vi "U3 PWM16.vi"(8 "error in":errorcluster, 9 "PWM Duty Cycle [%]":dbl=50.0 format="%.4f") -> (0 "error out":errorcluster)   [LabVIEW 2021]
panel:
  out "aTimerValues":u16[](array[numeric])
  in  "FirstFound":bool=TRUE
  in  "Address":string="1"
  out "Error Message":string
  # "Demonstrates 1 timer channel of 16-bit PWM output on FIO4 with a frequency of 40.7 Hz."
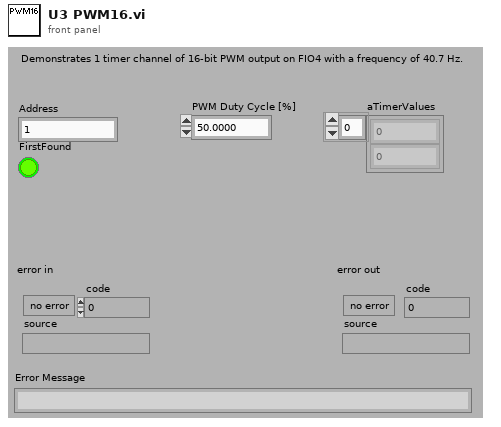
[diagram p1: front panel]
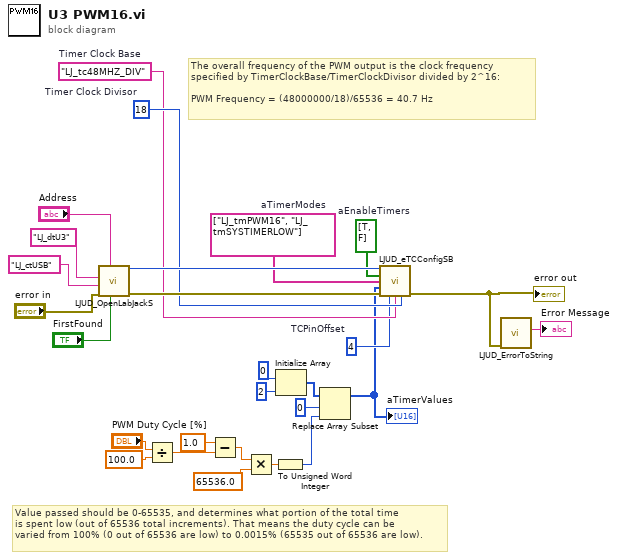
[diagram p0: block diagram]
diagram:
  w4 = 4  # TCPinOffset
  w3 = bool[] [TRUE, FALSE]  # aEnableTimers
  w6 = 18  # Timer Clock Divisor
  w5 = "LJ_tc48MHZ_DIV"  # Timer Clock Base
  w7 = string[] ["LJ_tmPWM16", "LJ_tmSYSTIMERLOW"]  # aTimerModes
  # "The overall frequency of the PWM output is the clock frequency\nspecified by TimerClockBase/TimerClockDivisor divided by 2^16:\n\nPWM Frequency = (48000000/18)/65536 = 40.7 Hz"
  # "Value passed should be 0-65535, and determines what portion of the total time\nis spent low (out of 65536 total increments). That means the duty cycle can be\nvaried from 100% (0 out of 65536 are low) to 0.0015% (65535 out of 65536 are low)."
  n1 = call "LJUD_OpenLabJackS.vi"("FirstFound"="FirstFound", "Address"="Address", "error in"="error in", "ConnectionType"="LJ_ctUSB", "DeviceType"="LJ_dtU3") -> ("error out"=w9:errorcluster, "Handle"=w8:i32)  [unwired: 4 in, 1 out]
  n2 = Divide(x="PWM Duty Cycle [%]", y=100.0) -> (x/y=w22:dbl)
  n3 = Subtract(x=1.0, y=w22) -> (x-y=w20:dbl)
  n4 = Multiply(x=w20, y=65536.0) -> (x*y=w11:dbl)
  n5 = To Unsigned Word Integer(number=w11) -> (unsigned 16bit integer=w10:u16)
  n6 = Initialize Array(u16 0 ("PWM Timer Value"), 2 ("Dimension Size")) -> (w15:u16[])
  n7 = Replace Array Subset(array=w15, new element=w10, index=0 ("Index")) -> (w1:u16[])
  "aTimerValues" <- w1
  n8 = call "LJUD_eTCConfigSB.vi"("Handle In"=w8, "aEnableTimers"=w3, "aTimerModes"=w7, "aTimerValues"=w1, "error in"=w9, "TCPinOffset"=w4, "TimerClockBase"=w5, "TimerClockDivisor"=w6) -> ("error out"=w2:errorcluster)  [unwired: 6 in, 1 out]
  "error out" <- w2
  n9 = call "LJUD_ErrorToString.vi"("error in"=w2) -> ("String"=→"Error Message":string)  [unwired: 10 in]
